vi "Write Send Data MSG.vi"(8 "error in (no error)":errorcluster, 10 "Controller.lvlib:Send Data Msg":refnum<class "Send Data Msg.lvclass">, 11 "Device in":refnum<class "Device.lvclass">) -> (0 "error out":errorcluster, 3 "Device out":refnum<class "Device.lvclass">)   [LabVIEW 2014, in "DAQ Device.lvlib" / "Device.lvclass"]
uses:
  Device.lvclass
  Messages/Send Data Msg.lvclass
  Device.lvclass/Device.ctl
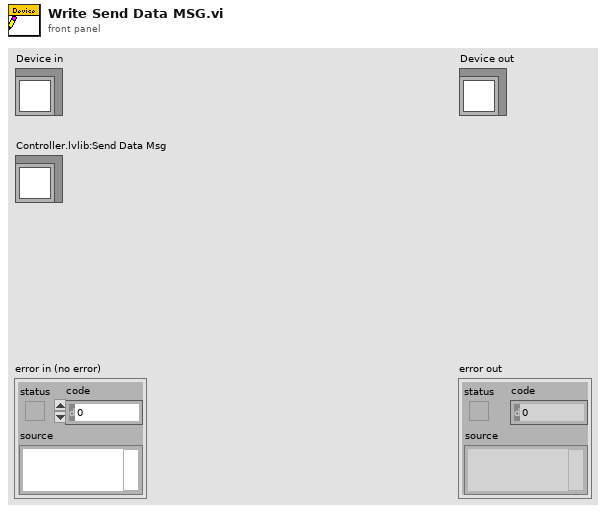
[diagram p1: front panel]
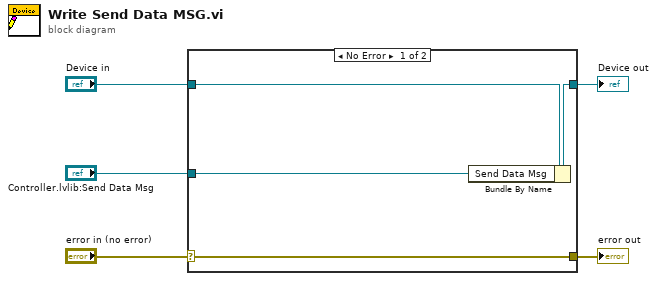
[diagram p0: block diagram]
diagram:
  n1 = case shown="No Error" "error in (no error)" {
    selector: "error in (no error)" -> [w9 w10]
    tunnel: [w9 w10] -> w4
    tunnel: [w7 w11] -> w2
    tunnel: "Device in" -> [w8 w11]
    tunnel: "Controller.lvlib:Send Data Msg" -> [w6 _]
    frame No Error {
      n2 = Bundle By Name(cluster=w8, "Send Data Msg"=w6) -> (w7:refnum<class "Device.lvclass">)
    }
    frame Error {
    }
  }
  "error out" <- w4
  "Device out" <- w2
